vi "LoadDemo.vi"(8 "error in (no error)":errorcluster, 10 "Engine in":refnum<class "Engine.lvclass">, 11 "AttractScreen in":refnum<class "AttractScreen.lvclass">) -> (0 "error out":errorcluster, 2 "Engine out":refnum<class "Engine.lvclass">, 3 "AttractScreen out":refnum<class "AttractScreen.lvclass">)   [LabVIEW 2019, in "RT_Game.lvlib" / "AttractScreen.lvclass"]
uses:
  AttractScreen.lvclass
  Engine/Engine.lvclass
  AttractScreen.lvclass/AttractScreen.ctl
  Engine/Engine.lvclass/Engine.ctl
  Engine/Write NextGame.vi
  Engine/Write SwitchGame_.vi
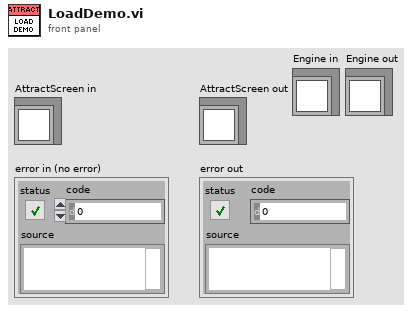
[diagram p1: front panel]
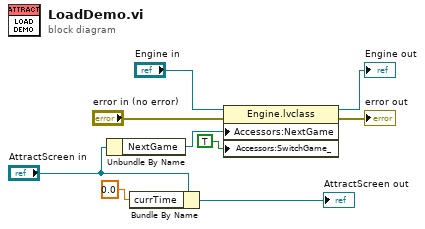
[diagram p0: block diagram]
diagram:
  n1 = Unbundle By Name("AttractScreen in") -> ("NextGame"=w1:refnum<class "Game.lvclass">)
  n2 = Bundle By Name(cluster="AttractScreen in", "currTime"=0.0) -> (→"AttractScreen out":refnum<class "AttractScreen.lvclass">)
  n3 = property class="Engine.lvclass"(reference="Engine in", error in="error in (no error)", "Accessors:NextGame"=w1, "Accessors:SwitchGame_"=TRUE ("SwitchGame_")) -> (reference out=→"Engine out":refnum<class "Engine.lvclass">, error out=→"error out":errorcluster)
